vi "Read Msg Input.vi"(10 "Msg Input":refnum<class "Msg Input.lvclass">) -> (4 "Teller":refnum<class "Teller.lvclass">)   [LabVIEW 2020, in "jettl.lvlib" / "Stopping jettl Msg.lvlib" / "Stopping Msg Input.lvlib"]
doc: "jettl 6.12.1.94\nNathan Davis - Nathan Davis\nCopyright (c) 2026, Nathan Davis\nMIT"
uses:
  Stopping Msg Input.lvlib
  Msg Input/Msg Input.lvclass
  Teller/Teller.lvclass
  Stopping Msg Input/Stopping Msg Input.lvclass
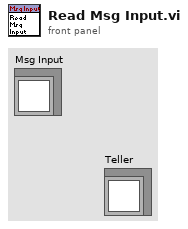
[diagram p1: front panel]
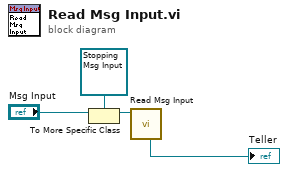
[diagram p0: block diagram]
diagram:
  n1 = To More Specific Class(target class=refnum<class "Stopping Msg Input.lvclass"> refnum ("_Template.lvlib:Templates.lvlib:TEMPLATE Msg.lvlib:TEMPLATE Msg Input.lvlib:TEMPLATE Msg Input.lvclass"), reference="Msg Input") -> (specific class reference=w3:refnum<class "Stopping Msg Input.lvclass">)  [unwired: 1 in, 1 out]
  n2 = call "Read Msg Input.vi"("Stopping Msg Input in"=w3) -> ("Teller"=→"Teller":refnum<class "Teller.lvclass">)  [unwired: 10 in]
